vi "OldStageController.vi"() -> ()   [LabVIEW 2013]
panel:
  in  "motorSpeed":dbl caption="Motor Speed" min=0.0 max=2000.0 format="%#.4g"
  in  "setEncodertoZero":bool caption="Set Encoder to Zero"
  in  "home":bool caption="Home"
  in  "Motor COM Port":refnum<visa-resource-name>="COM4"
  in  "Encoder COM Port":refnum<visa-resource-name>="COM1"
  in  "showTerminal":bool caption="Show Terminal"
  in  "EXIT":bool
  out "currentPos":dbl caption="Current Position (mm)" format="%.3g"
  in  "goToPos3":bool caption="Go to Position 3"
  in  "goToPos2":bool caption="Go to Position 2"
  in  "goToPos1":bool caption="Go to Position 1"
  in  "pos3":dbl=1.0 caption="Position 3 (mm)" min=1.0 max=4060.0 format="%.3g"
  in  "pos2":dbl caption="Position 2 (mm)" min=1.0 max=4060.0 format="%.3g"
  in  "pos1":dbl=1.0 caption="Position 1 (mm)" min=1.0 max=4060.0 format="%.3g"
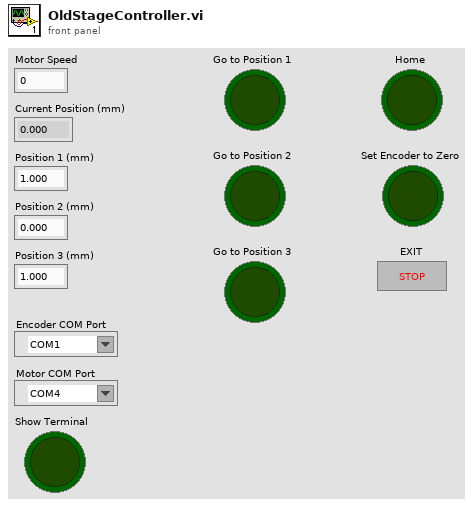
[diagram p1: front panel]
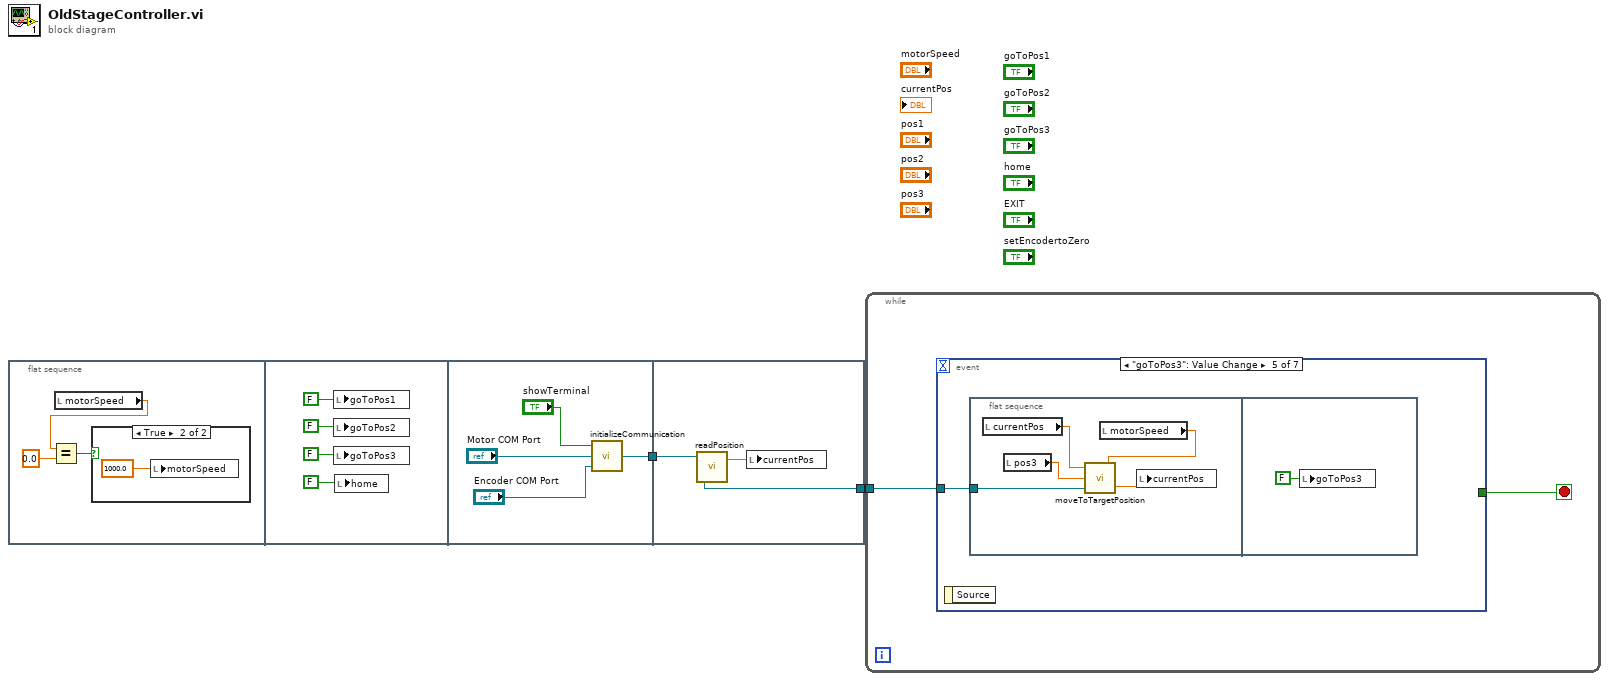
[diagram p0: block diagram]
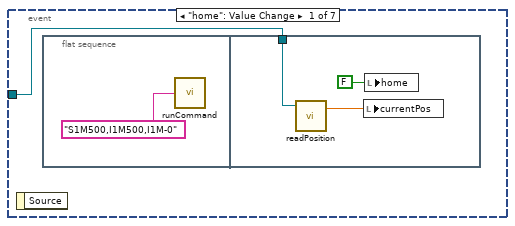
[diagram p3: hidden frame]
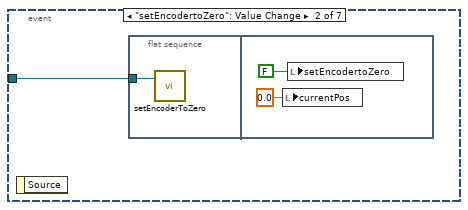
[diagram p4: hidden frame]
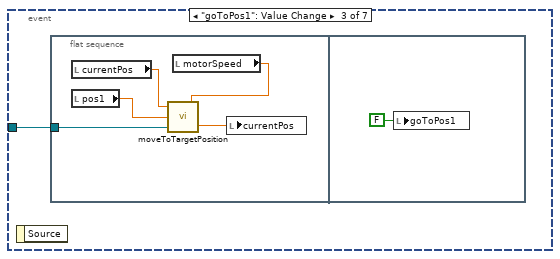
[diagram p5: hidden frame]
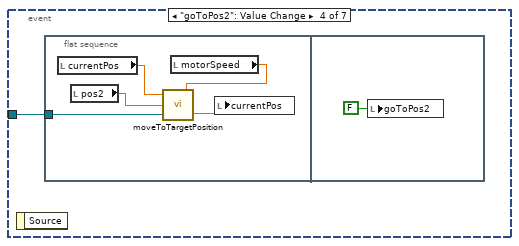
[diagram p6: hidden frame]
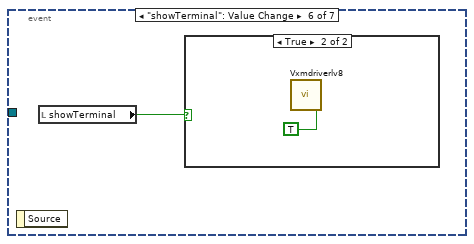
[diagram p7: hidden frame]
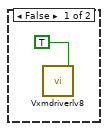
[diagram p8: hidden frame]
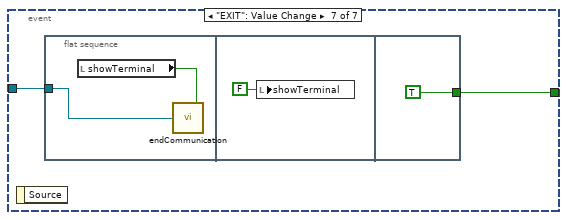
[diagram p9: hidden frame]
diagram:
  n1 = flat-sequence {
    tunnel: [w11] -> w2
    tunnel: w2 -> [w17]
    tunnel: [w16] -> w1
    frame #0 {
      n2 = local read "motorSpeed"() -> (w5:dbl)
      n3 = Equal?(x=w5, y=0.0) -> (x = y?=w3:bool)
      n4 = case shown="True" w3 {
        frame False {
        }
        frame True {
          n5 = local write "motorSpeed"(1000.0 ("Motor Speed")) -> ()
        }
      }
    }
    frame #1 {
      n6 = local write "goToPos1"(FALSE ("goToPos1")) -> ()
      n7 = local write "goToPos2"(FALSE ("goToPos2")) -> ()
      n8 = local write "goToPos3"(FALSE ("goToPos3")) -> ()
      n9 = local write "home"(FALSE ("Home")) -> ()
    }
    frame #2 {
      n10 = call "initializeCommunication.vi"("Encoder COM Port"="Encoder COM Port", "Motor COM Port"="Motor COM Port", "Show Terminal"="showTerminal") -> ("Encoder VISA Resource Name (out)"=w11:refnum<visa-resource-name>)
    }
    frame #3 {
      n11 = call "readPosition.vi"("VISA resource name"=w17) -> ("position"=w15:dbl, "VISA resource name out"=w16:refnum<visa-resource-name>)  [unwired: 1 in, 1 out]
      n12 = local write "currentPos"(w15) -> ()
    }
  }
  n13 = while {
    tunnel: w1 -> [w19]
    stop <- w18 stop-if-true
    n14 = event shown="[4] \"goToPos3\": Value Change" {
      selector: _ -> [_ _ _ _ _ _ _]
      dyn-events: _ -> [_ _ _ _ _ _ _]
      timeout: _ -> [_ _ _ _ _ _ _]
      tunnel: w19 -> [w20 w25 w29 w36 w43 _ w54]
      tunnel: [_ _ _ _ _ _ w53] -> w18
      event "home": Value Change {
        n15 = event-data() -> ()  [unwired: 1 in, 1 out]
        n16 = flat-sequence {
          tunnel: w20 -> [w22]
          frame #0 {
            n17 = call "runCommand.vi"("command"="S1M500,I1M500,I1M-0") -> ()  [unwired: 1 in]
          }
          frame #1 {
            n18 = call "readPosition.vi"("VISA resource name"=w22) -> ("position"=w23:dbl)  [unwired: 1 in, 2 out]
            n19 = local write "currentPos"(w23) -> ()
            n20 = local write "home"(FALSE ("Home")) -> ()
          }
        }
      }
      event "setEncodertoZero": Value Change {
        n21 = event-data() -> ()  [unwired: 1 in, 1 out]
        n22 = flat-sequence {
          tunnel: w25 -> [w26]
          frame #0 {
            n23 = call "setEncoderToZero.vi"("VISA resource name"=w26) -> ()  [unwired: 1 in, 2 out]
          }
          frame #1 {
            n24 = local write "currentPos"(0.0 ("currentPos")) -> ()
            n25 = local write "setEncodertoZero"(FALSE ("Set Encoder to Zero")) -> ()
          }
        }
      }
      event "goToPos1": Value Change {
        n26 = event-data() -> ()  [unwired: 1 in, 1 out]
        n27 = flat-sequence {
          tunnel: w29 -> [w34]
          frame #0 {
            n28 = local read "currentPos"() -> (w32:dbl)
            n29 = local read "pos1"() -> (w33:dbl)
            n30 = local read "motorSpeed"() -> (w30:dbl)
            n31 = call "moveToTargetPosition.vi"("speed"=w30, "Encoder COM Port"=w34, "targetPos"=w33, "currentPos"=w32) -> ("updatedCurrentPos"=w31:dbl)
            n32 = local write "currentPos"(w31) -> ()
          }
          frame #1 {
            n33 = local write "goToPos1"(FALSE ("goToPos1")) -> ()
          }
        }
      }
      event "goToPos2": Value Change {
        n34 = event-data() -> ()  [unwired: 1 in, 1 out]
        n35 = flat-sequence {
          tunnel: w36 -> [w41]
          frame #0 {
            n36 = local read "currentPos"() -> (w40:dbl)
            n37 = local read "pos2"() -> (w39:dbl)
            n38 = local read "motorSpeed"() -> (w37:dbl)
            n39 = call "moveToTargetPosition.vi"("speed"=w37, "Encoder COM Port"=w41, "targetPos"=w39, "currentPos"=w40) -> ("updatedCurrentPos"=w38:dbl)
            n40 = local write "currentPos"(w38) -> ()
          }
          frame #1 {
            n41 = local write "goToPos2"(FALSE ("goToPos2")) -> ()
          }
        }
      }
      event "goToPos3": Value Change {
        n42 = event-data() -> ()  [unwired: 1 in, 1 out]
        n43 = flat-sequence {
          tunnel: w43 -> [w47]
          frame #0 {
            n44 = local read "currentPos"() -> (w46:dbl)
            n45 = local read "pos3"() -> (w48:dbl)
            n46 = local read "motorSpeed"() -> (w44:dbl)
            n47 = call "moveToTargetPosition.vi"("speed"=w44, "Encoder COM Port"=w47, "targetPos"=w48, "currentPos"=w46) -> ("updatedCurrentPos"=w45:dbl)
            n48 = local write "currentPos"(w45) -> ()
          }
          frame #1 {
            n49 = local write "goToPos3"(FALSE ("goToPos3")) -> ()
          }
        }
      }
      event "showTerminal": Value Change {
        n50 = event-data() -> ()  [unwired: 1 in, 1 out]
        n51 = local read "showTerminal"() -> (w50:bool)
        n52 = case shown="True" w50 {
          frame False {
            n53 = call "Vxmdriverlv8.Vi"("Hide Terminal"=TRUE) -> ()  [unwired: 21 in, 6 out]
          }
          frame True {
            n54 = call "Vxmdriverlv8.Vi"("Show Terminal"=TRUE) -> ()  [unwired: 21 in, 6 out]
          }
        }
      }
      event "EXIT": Value Change {
        n55 = event-data() -> ()  [unwired: 1 in, 1 out]
        n56 = flat-sequence {
          tunnel: w54 -> [w56]
          tunnel: [TRUE] -> w53
          frame #0 {
            n57 = local read "showTerminal"() -> (w55:bool)
            n58 = call "endCommunication.vi"("Show Terminal"=w55, "Encoder COM Port"=w56) -> ()
          }
          frame #1 {
            n59 = local write "showTerminal"(FALSE ("Show Terminal")) -> ()
          }
          frame #2 {
          }
        }
      }
    }
  }
